vi "Read Pin.vi"(6 "Pin":u16, 8 "error in (no error)":errorcluster, 9 "Port":u16, 10 "VISA resource name":refnum<visa-resource-name>, 11 "Cypress in":refnum<class "Cypress.lvclass">) -> (0 "error out":errorcluster, 1 "Boolean":bool, 2 "VISA resource name 2":refnum<visa-resource-name>, 3 "Cypress out":refnum<class "Cypress.lvclass">)   [LabVIEW 2020, in "Cypress.lvclass"]
uses:
  Cypress.lvclass
  Abstract/Serial Device/Serial Device.lvclass
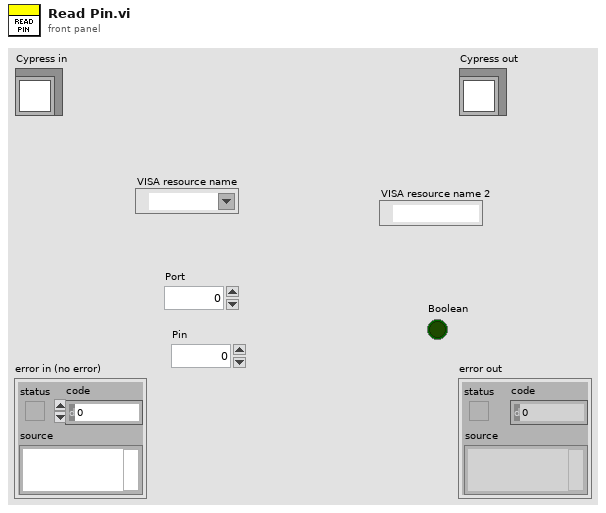
[diagram p1: front panel]
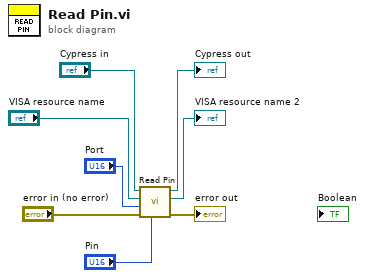
[diagram p0: block diagram]
diagram:
  n1 = call-parent "Read Pin.vi"("Pin"="Pin", "error in (no error)"="error in (no error)", "Port"="Port", "VISA resource name"="VISA resource name", "Serial Device in"="Cypress in") -> ("error out"=→"error out":errorcluster, "VISA resource name 2"=→"VISA resource name 2":refnum<visa-resource-name>, "Serial Device out"=→"Cypress out":refnum<class "Cypress.lvclass">)  [unwired: 3 in, 1 out]
